vi "Terminal_Control_Poly.vi"   [LabVIEW 2012]
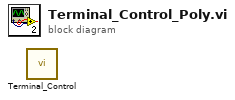
[diagram p0: block diagram]
diagram:
  n1 = call "Terminal_Control.vi"() -> ()  [unwired: 11 in, 1 out]
